vi "ROI grp-Event handler-Groups button press.vi"(11 "Groups window notifier":refnum<notifier>) -> ()   [LabVIEW 2020]
uses:
  Typedefs/ROI grp-process states enum.ctl
  Globals/gl_ROI grp window globals.vi
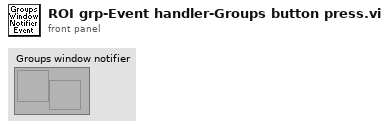
[diagram p1: front panel]
types:
  T1 = typedef "ROI grp-process states enum.ctl" = enum16{"Open window", "Stop loop"}
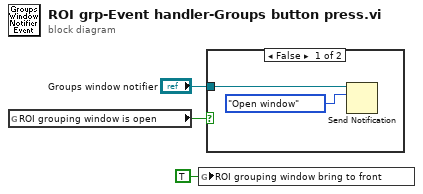
[diagram p0: block diagram]
diagram:
  n1 = global read "gl_ROI grp window globals.vi" "ROI grouping window is open"() -> (w2:bool)
  n2 = global write "gl_ROI grp window globals.vi" "ROI grouping window bring to front"(TRUE ("Bring POI grouping window to front")) -> ()
  n3 = case shown="False" w2 {
    tunnel: "Groups window notifier" -> [w5 _]
    frame False {
      n4 = Send Notification(notification=ROI_grp-process_states_enum."Open window" ("Function"), notifier=w5) -> ()  [unwired: 1 in, 2 out]
    }
    frame True {
    }
  }
